vi "FWHM of chosen peak in array.vi"(6 "0.5 means FWHM":dbl=0.5 format="%#_13g", 9 "amplitude of peak":dbl, 10 "index of peak":dbl, 11 "counts":dbl[](graph)) -> (1 "width of peak higher side":dbl, 2 "FWHM":dbl, 3 "width peak lower side":dbl)   [LabVIEW 2020]
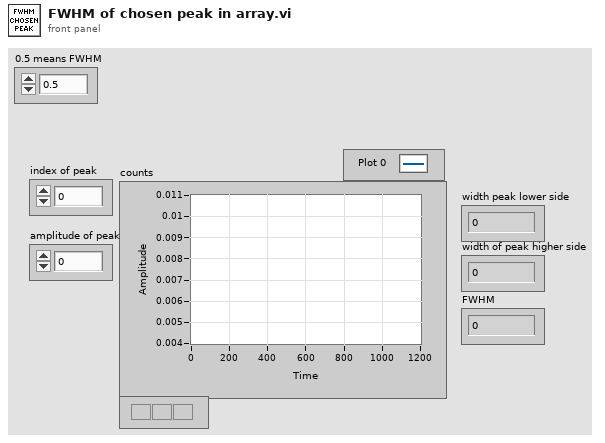
[diagram p1: front panel]
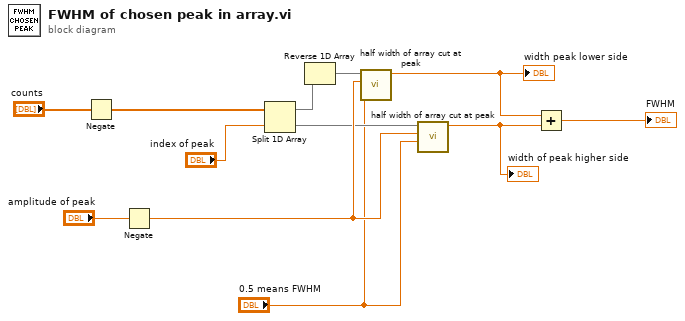
[diagram p0: block diagram]
diagram:
  n1 = Negate(x="counts") -> (-x=w6:dbl[])
  n2 = Negate(x="amplitude of peak") -> (-x=w5:dbl)
  n3 = Split 1D Array(array=w6, index="index of peak") -> (first subarray=w4:dbl[], second subarray=w2:dbl[])
  n4 = Reverse 1D Array(array=w4) -> (reversed array=w3:dbl[])
  n5 = call "half width of array cut at peak.vi"("0.5 means FWHM"="0.5 means FWHM", "amplitude value biggest peak"=w5, "counts"=w3) -> ("half width half max"=w10:dbl)  [unwired: 8 in]
  "width peak lower side" <- w10
  n6 = call "half width of array cut at peak.vi"("0.5 means FWHM"="0.5 means FWHM", "amplitude value biggest peak"=w5, "counts"=w2) -> ("half width half max"=w11:dbl)  [unwired: 8 in]
  "width of peak higher side" <- w11
  n7 = Add(x=w10, y=w11) -> (x+y=→"FWHM":dbl)
